vi "evaluate_waveforms.vi"(8 "error in (no error)":errorcluster, 10 "ExperimentVariables (in)":refnum<class "ExperimentVariables.lvclass">, 11 "HSDIO (in)":refnum<class "HSDIO.lvclass">) -> (0 "error out":errorcluster, 1 "final script":string, 2 "A waveform was padded":bool, 3 "HSDIO instrument handle":refnum<k15>, 4 "waveform names":string[](array[string]), 5 "HSDIO Status":T1={"Channel List"="0,1,3,4,5", "Loaded Waveforms"=["Hex_Array_Loading"], "A waveform was padded"=FALSE, "final script this iteration"="script script1\r\nGenerate w00000000\r\nWait 49999\nGenerate w00000200\r\nWait 49999\nGenerate w00000000\r\nWait 49999\nGenerate w00000000\r\nWait 849999\nGenerate w80000000\r\nWait 559999\nGenerate w80000008\r\nWait 439999\nGenerate wD000001A\r\nWait 59999\nGenerate wB0000019\r\nWait 499999\nGenerate w30000011\r\nWait 499999\nGenerate w50000012\r\nWait 1999999\nGenerate w30000031\r\nWait 999999\nGenerate w30000011\r\nWait 8999999\nGenerate w10000010\r\nWait 6939998\nGenerate w10000010\r\nGenerate w00000000\r\nend script\r\n"})   [LabVIEW 2013]
doc: "1. Re-evaluate all the waveforms for the current values of the variables.\n2. Upload the waveforms.\n3. For each measurement\n a. Run the previously loaded script\n b. Wait until the script completes\n c. Acquire images\n4. Remove waveforms from memory"
uses:
  <vilib>/regexp/Match Regular Expression.xnode
  <instrlib>/niHSDIO/niHSDIO.llb/niHSDIO Write Named Waveform (1D U32).vi
  HSDIO/HSDIO.lvclass
  ExperimentVariables/ExperimentVariables.lvclass
panel:
  out "HSDIO":refnum<class "HSDIO.lvclass">
  out "ExperimentVariables":refnum<class "ExperimentVariables.lvclass">
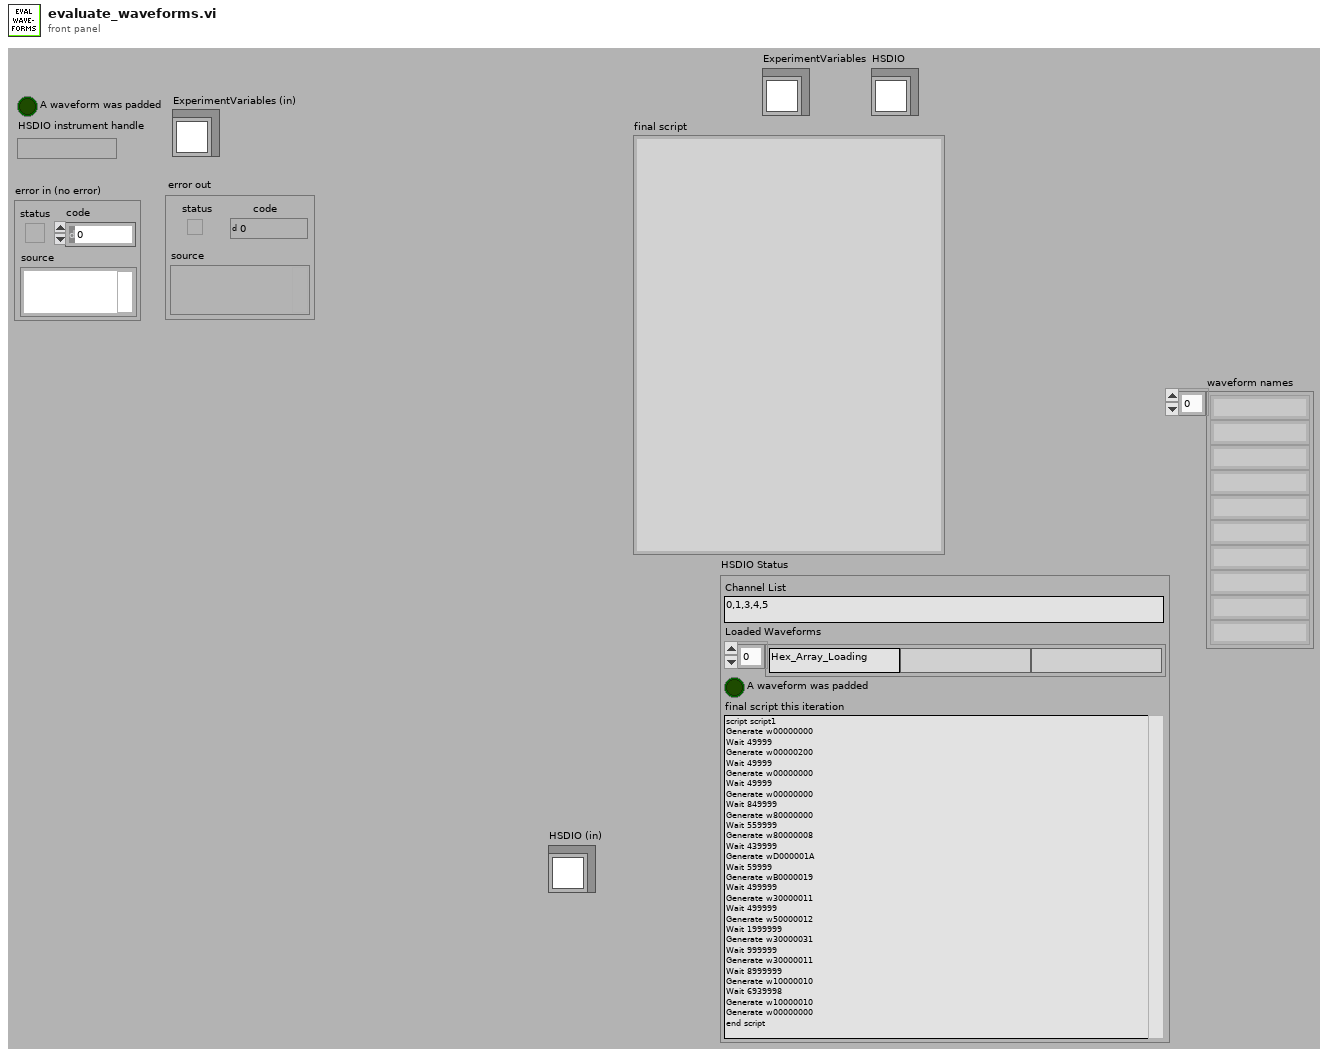
[diagram p1: front panel]
types:
  T1 = cluster{"Channel List":string, "Loaded Waveforms":string[], "A waveform was padded":bool, "final script this iteration":string}
  T2 = typedef "HSDIO.lvclass/HSDIO_settings.ctl" = cluster{"Enable HSDIO Pulses":bool, "Resource Name":refnum<k15>, "Clock Rate":dbl, "Array of Script Triggers":cluster{"trigger id (script trigger 0)":T3, "source (PFI 0)":T4, "Trigger Type":enum32{"Edge", "Level"}, "edge":T5, "level":T6}[], "Pulse Generation Script":string, "Start Trigger":cluster{"Wait for start trigger?":bool, "source (PFI 0)":T4, "edge (rising)":T5, "description":string}, "Hardware alignment quantum\n(in samples)":u16, "Inital State":string, "Idle State":string, "Active Channels":string, "Array of Waveforms":T7[], "description":string}
  T3 = typedef "niHSDIO_ctl Trigger Script - trigID Values (Ring).ctl" = string
  T4 = typedef "niHSDIO_ctl Trigger Source Values (Ring).ctl" = string
  T5 = typedef "niHSDIO_ctl Trigger DigEdge - Edge Values (Ring).ctl" = i32
  T6 = typedef "niHSDIO_ctl Trigger DigLvl - Level Values (Ring).ctl" = i32
  T7 = typedef "HSDIO.lvclass/waveform.ctl" = cluster{"name":string, "transitions":u32[], "states":u8[][]}
  T8 = cluster{"trigger id (script trigger 0)":T3, "source (PFI 0)":T4, "Trigger Type":enum32{"Edge", "Level"}, "edge":T5, "level":T6}[]
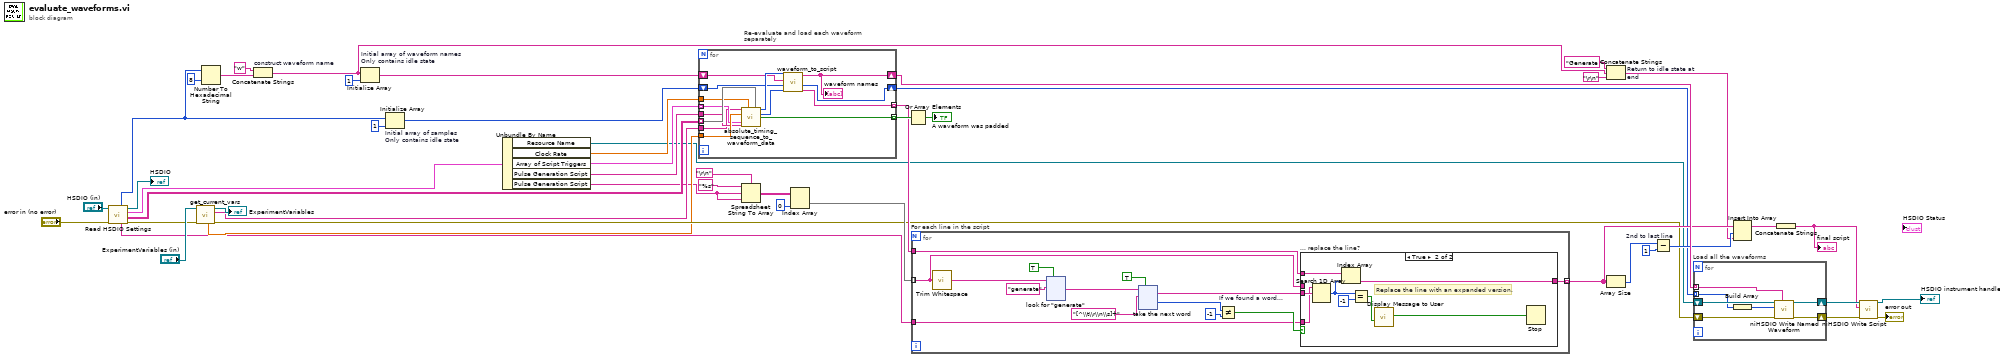
[diagram p0: block diagram]
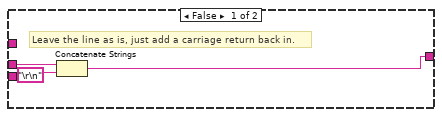
[diagram p2: hidden frame]
diagram:
  n1 = call-dynamic "Read HSDIO Settings.vi"("error in (no error)"="error in (no error)", "HSDIO in"="HSDIO (in)") -> ("error out"=w15:errorcluster, "array of waveforms"=w7:string[][][], "HSDIO Settings"=w12:T2, "HSDIO out"=→"HSDIO":refnum<class "HSDIO.lvclass">, "waveform names"=w6:string[], "Idle State (Binary)"=w2:u32)  [unwired: 4 in]
  n2 = call-dynamic "get_current_vars.vi"("error in (no error)"=w15, "ExperimentVariables in"="ExperimentVariables (in)") -> ("error out"=w13:errorcluster, "variables and parameter names"=w8:string[], "ExperimentVariables out"=→"ExperimentVariables":refnum<class "ExperimentVariables.lvclass">, "current variable and parameter values"=w9:dbl[])  [unwired: 4 in, 2 out]
  n3 = Number To Hexadecimal String(1:i16 8 ("width (-)"), 2:w2) -> (0:w32:string)
  n4 = Concatenate Strings "construct waveform name"("w" ("string"), w32) -> (w28:string)
  n5 = Initialize Array "Initial array of waveform names\nOnly contains idle state"(w28, 1 ("dimension size")) -> (w30:string[])
  n6 = Initialize Array "Initial array of samples\nOnly contains idle state"(w2, 1 ("dimension size")) -> (w35:u32[])
  n7 = Unbundle By Name(w12) -> ("Resource Name"=w1:refnum<k15>, "Clock Rate"=w10:dbl, "Array of Script Triggers"=w5:T8, "Pulse Generation Script"=w4:string, "Pulse Generation Script"=w3:string)
  n8 = for "Re-evaluate and load each waveform separately" {
    tunnel: w7 -> [w63] mode=indexing
    tunnel: w9 -> [w62]
    tunnel: w8 -> [w57]
    tunnel: w10 -> [w61]
    tunnel: [w60] -> w49 mode=indexing
    tunnel: w4 -> [w59]
    tunnel: w5 -> [w58] mode=indexing
    tunnel: [w51] -> w42 mode=indexing
    shift-right: [w54] -> w37
    shift-left: w30 -> [w55]
    shift-right: [w50] -> w19
    shift-left: w35 -> [w52]
    n9 = call "absolute_timing_sequence_to_waveform_data.vi"("Variable Names"=w57, "Clock Rate"=w61, "Timing Sequence Control (ms)"=w63, "Current Value Array"=w62, "Force waveform length to be multiple of 2\n(Necessary on old hardware)"=w59, "units/sec (ms=1000)"=w58) -> ("Transitions"=w56:u32[], "Data"=w53:u32[], "Waveform was padded"=w60:bool)  [unwired: 5 in, 2 out]
    n10 = call "waveform_to_script.vi"("Data"=w53, "existing waveform samples (in)"=w52, "existing waveform names"=w55, "Transitions (sorted and reduced)"=w56) -> ("script"=w51:string, "waveform samples (out)"=w50:u32[], "waveform names"=w54:string[])  [unwired: 4 in, 1 out]
    "waveform names" <- w54
  }
  n11 = Spreadsheet String To Array(delimiter (Tab)="\r\n", format string="%s", spreadsheet string=w3, array type (2D Dbl)=w3) -> (array=w41:string[][])
  n12 = Index Array(array=w41, index (col)=0 ("index (row)")) -> (element=w43:string[])  [unwired: 1 in]
  n13 = Or Array Elements(Boolean array=w49) -> (logical OR=→"A waveform was padded":bool)
  n14 = for "For each line in the script" {
    tunnel: w43 -> [w64] mode=indexing
    tunnel: w42 -> [w66]
    tunnel: w6 -> [w68]
    tunnel: [w67] -> w26 mode=indexing
    n15 = call <vilib>:"Trim Whitespace.vi"("string"=w64) -> ("trimmed string"=w76:string)  [unwired: 1 in]
    n16 = xnode "look for \"generate\""("input string"=w76, "regular expression"="generate", "ignore case? (F)"=TRUE) -> ("after match"=w72:string)  [unwired: 3 in, 4 out]
    n17 = xnode "take the next word"("input string"=w72, "regular expression"="[^\\t\\r\\n\\s]+", "ignore case? (F)"=TRUE) -> ("whole match"=w70:string, "offset past match"=w71:i32)  [unwired: 3 in, 3 out]
    n18 = Not Equal? "If we found a word..."(x=w71, y=-1) -> (x != y?=w69:bool)
    n19 = case "... replace the line?" shown="True" w69 {
      tunnel: w70 -> [_ w88]
      tunnel: [w78 w81] -> w67
      tunnel: w64 -> [w80 _]
      tunnel: w66 -> [_ w82]
      tunnel: w68 -> [_ w87]
      frame False {
        # "Leave the line as is, just add a carriage return back in."
        n20 = Concatenate Strings(w80, "\r\n") -> (w78:string)
      }
      frame True {
        # "Replace the line with an expanded version."
        n21 = Search 1D Array(1D array=w87, element=w88) -> (index of element=w83:i32)  [unwired: 1 in]
        n22 = Index Array(array=w82, index=w83) -> (element=w81:string)
        n23 = Equal?(x=w83, y=-1) -> (x = y?=w85:bool)
        n24 = call "Display Message to User"("Enable"=w85) -> ("OK"=w84:bool)  [unwired: 9 in, 1 out]
        n25 = Stop(stop? (T)=w84) -> ()
      }
    }
  }
  n26 = Concatenate Strings "Return to idle state at end"("Generate " ("string"), w28, "\r\n") -> (w22:string)
  n27 = Array Size(array=w26) -> (size(s)=w25:i32)
  n28 = Subtract "2nd to last line"(x=w25, y=1) -> (x-y=w23:i32)
  n29 = for "Load all the waveforms" {
    tunnel: w37 -> [w313] mode=indexing
    shift-right: [w316] -> w38
    shift-left: w1 -> [w317]
    shift-right: [w314] -> w39
    shift-left: w13 -> [w315]
    tunnel: w19 -> [w312] mode=indexing
    n30 = Build Array(w312) -> (w311:u32[])
    n31 = call-poly <instrlib>:"niHSDIO Write Named Waveform.vi"("waveform name (default:\"\")"=w313, "error in (no error)"=w315, "data"=w311, "instrument handle"=w317) -> ("error out"=w314:errorcluster, "instrument handle out"=w316:refnum<k15>)  [unwired: 6 in]
  }
  n32 = Insert Into Array(array=w26, index=w23, new element=w22) -> (w21:string[])
  n33 = Concatenate Strings(w21) -> (w20:string)
  "final script" <- w20
  n34 = call <instrlib>:"niHSDIO Write Script.vi"("error in (no error)"=w39, "script"=w20, "instrument handle"=w38) -> ("error out"=→"error out":errorcluster, "instrument handle out"=→"HSDIO instrument handle":refnum<k15>)  [unwired: 7 in]
